vi "command_damn_yankee.vi"(6 "Dynamixel Bounds":T1, 7 "VISA Refnum in":refnum<visa-resource-name>, 8 "error in (no error)":errorcluster, 9 "Rudder Control":dbl, 10 "Sail Control":T4 {"MainSailSuggestion" min=0.0 max=1.0; "JibSailSuggestion" min=0.0 max=1.0}, 11 "Dynamixel Cycles":T3) -> (0 "error out":errorcluster, 1 "Rudder written value":dbl, 2 "Jib written value":dbl, 3 "Main written value":dbl, 5 "VISA Refnum out":refnum<visa-resource-name>)   [LabVIEW 2013]
doc: "This code takes a series of setpoints and the necessary corresponding information (cycle #, bounds) to set the motors. It is hard-coded right now for 0, 1, and 2 to be the rudder, sail, and sail motors."
uses:
  Data/TypeDefs/Sail Set Suggestions.ctl
  Data/TypeDefs/DynamixelCycleTracker.ctl
  Data/TypeDefs/MotorSetup.ctl
  Data/TypeDefs/DynamixelSetupInfo.ctl
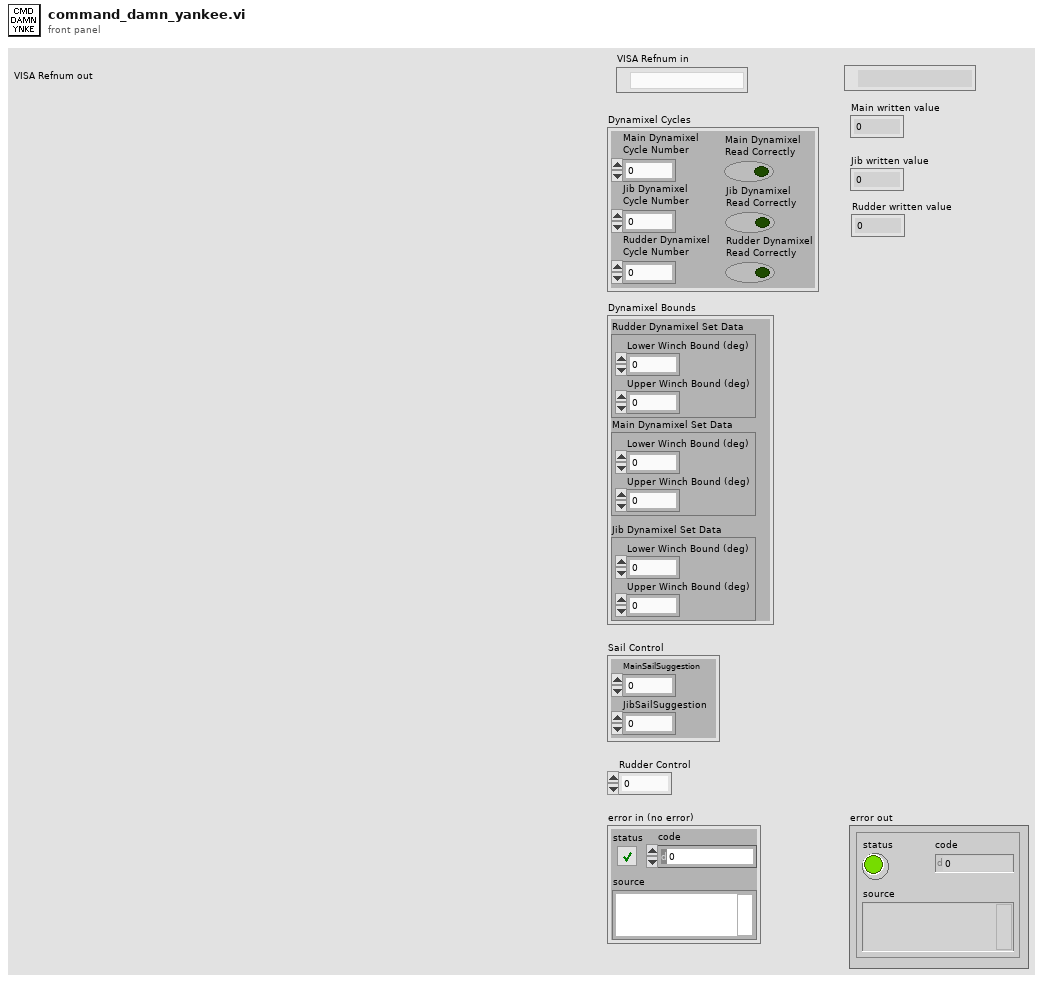
[diagram p1: front panel]
types:
  T1 = typedef "MotorSetup.ctl" = cluster{"Main Dynamixel Set Data":T2, "Rudder Dynamixel Set Data":T2, "Jib Dynamixel Set Data":T2}
  T2 = typedef "DynamixelSetupInfo.ctl" = cluster{"Lower Winch Bound (deg)":dbl, "Upper Winch Bound (deg)":dbl}
  T3 = typedef "DynamixelCycleTracker.ctl" = cluster{"Main Dynamixel\nCycle Number":i32, "Jib Dynamixel\nCycle Number":i32, "Rudder Dynamixel\nCycle Number":i32, "Main Dynamixel\nRead Correctly":bool, "Jib Dynamixel\nRead Correctly":bool, "Rudder Dynamixel\nRead Correctly":bool}
  T4 = typedef "Sail Set Suggestions.ctl" = cluster{"MainSailSuggestion":dbl, "JibSailSuggestion":dbl}
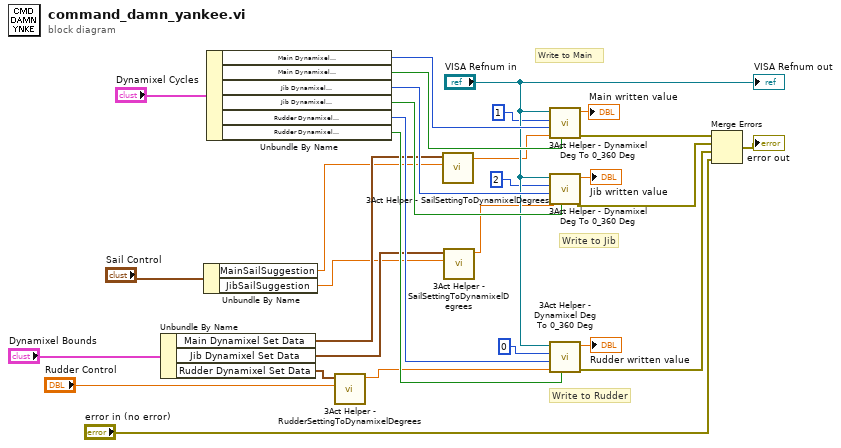
[diagram p0: block diagram]
diagram:
  # "Write to Rudder"
  # "Write to Jib"
  # "Write to Main"
  n1 = Unbundle By Name("Dynamixel Bounds") -> ("Main Dynamixel Set Data"=w10:T2, "Jib Dynamixel Set Data"=w15:T2, "Rudder Dynamixel Set Data"=w9:T2)
  n2 = Unbundle By Name("Sail Control") -> ("MainSailSuggestion"=w1:dbl, "JibSailSuggestion"=w2:dbl)
  n3 = Unbundle By Name("Dynamixel Cycles") -> ("Main Dynamixel\nCycle Number"=w17:i32, "Main Dynamixel\nRead Correctly"=w25:bool, "Jib Dynamixel\nCycle Number"=w24:i32, "Jib Dynamixel\nRead Correctly"=w26:bool, "Rudder Dynamixel\nCycle Number"=w23:i32, "Rudder Dynamixel\nRead Correctly"=w27:bool)
  n4 = call "3Act Helper - RudderSettingToDynamixelDegrees.vi"("Suggested Rudder Setpoint"="Rudder Control", "Dynamixel Set Data"=w9) -> ("Dynamixel Angle"=w22:dbl)  [unwired: 9 in]
  n5 = call "3Act Helper - SailSettingToDynamixelDegrees.vi"("SailSuggestion"=w1, "Dynamixel Set Data"=w10) -> ("Dynamixel Angle"=w6:dbl)  [unwired: 9 in]
  n6 = call "3Act Helper - SailSettingToDynamixelDegrees.vi"("SailSuggestion"=w2, "Dynamixel Set Data"=w15) -> ("Dynamixel Angle"=w7:dbl)  [unwired: 9 in]
  n7 = call "3Act Helper - Dynamixel Deg To 0_360 Deg.vi"("Motor Read\nCorrectly"=w25, "Dynamixel Setpoint In (deg)"=w6, "Dynamixel Cycle Number"=w17, "Motor ID"=u8 1 ("Motor ID (0)"), "VISA resource name"="VISA Refnum in") -> ("Error out"=w11:errorcluster, "Written value"=→"Main written value":dbl)  [unwired: 4 in, 1 out]
  n8 = call "3Act Helper - Dynamixel Deg To 0_360 Deg.vi"("Motor Read\nCorrectly"=w26, "Dynamixel Setpoint In (deg)"=w7, "Dynamixel Cycle Number"=w24, "Motor ID"=u8 2 ("Motor ID (0)"), "VISA resource name"="VISA Refnum in") -> ("Error out"=w12:errorcluster, "Written value"=→"Jib written value":dbl)  [unwired: 4 in, 1 out]
  n9 = call "3Act Helper - Dynamixel Deg To 0_360 Deg.vi"("Motor Read\nCorrectly"=w27, "Dynamixel Setpoint In (deg)"=w22, "Dynamixel Cycle Number"=w23, "Motor ID"=u8 0 ("Motor ID (0)"), "VISA resource name"="VISA Refnum in") -> ("Error out"=w13:errorcluster, "Written value"=→"Rudder written value":dbl)  [unwired: 4 in, 1 out]
  n10 = Merge Errors(w11, w12, w13, "error in (no error)") -> (→"error out":errorcluster)
  "VISA Refnum out" <- "VISA Refnum in"
